vi "Read Step UI Main VI Ref.vi"(8 "error in (no error)":errorcluster, 11 "Step UI in":refnum<class "Step UI.lvclass">) -> (0 "error out":errorcluster, 2 "Step UI Main VI Ref":refnum<vi>, 3 "Step UI out":refnum<class "Step UI.lvclass">)   [LabVIEW 2015, in "Step UI.lvclass"]
uses:
  Step UI.lvclass
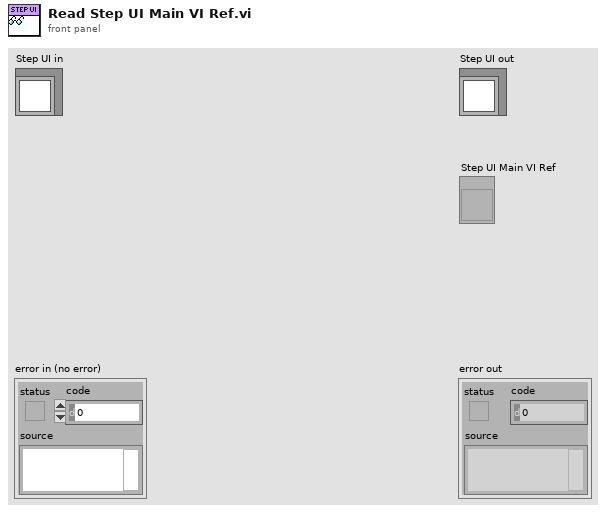
[diagram p1: front panel]
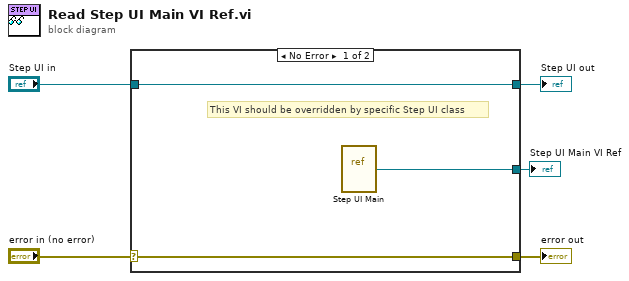
[diagram p0: block diagram]
diagram:
  n1 = case shown="No Error" "error in (no error)" {
    selector: "error in (no error)" -> [w8 w9]
    tunnel: [w8 w9] -> w4
    tunnel: [w7 w10] -> w2
    tunnel: "Step UI in" -> [w7 w10]
    tunnel: [w6 _] -> w1
    frame No Error {
      # "This VI should be overridden by specific Step UI class"
      n2 = vi-ref "Step UI Main.vi"() -> (w6:refnum<vi>)
    }
    frame Error {
    }
  }
  "error out" <- w4
  "Step UI out" <- w2
  "Step UI Main VI Ref" <- w1
